vi "Create Init File.vi"(8 "error in (no error)":errorcluster caption="entrée d'erreur (pas d'erreur)", 9 "Nom du fichier ini":string, 10 "Répertoire de l'appli":path, 11 "Container en entrée":refnum<class "Container.lvclass">) -> (0 "error out":errorcluster caption="sortie d'erreur", 2 "Répertoire fichier ini out":path, 3 "Container en sortie":refnum<class "Container.lvclass">)   [LabVIEW 2023, in "Container.lvclass"]
uses:
  Container.lvclass
  Container.lvclass/Container.ctl
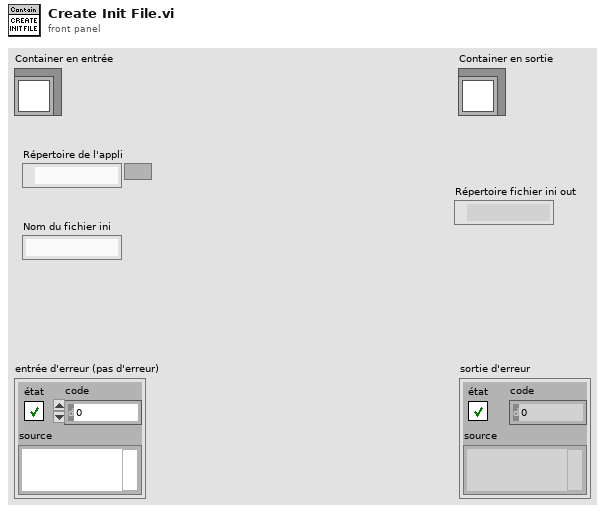
[diagram p1: front panel]
types:
  T1 = enum16{"open", "replace", "create", "open or create", "replace or create", "replace or create with confirmation"}
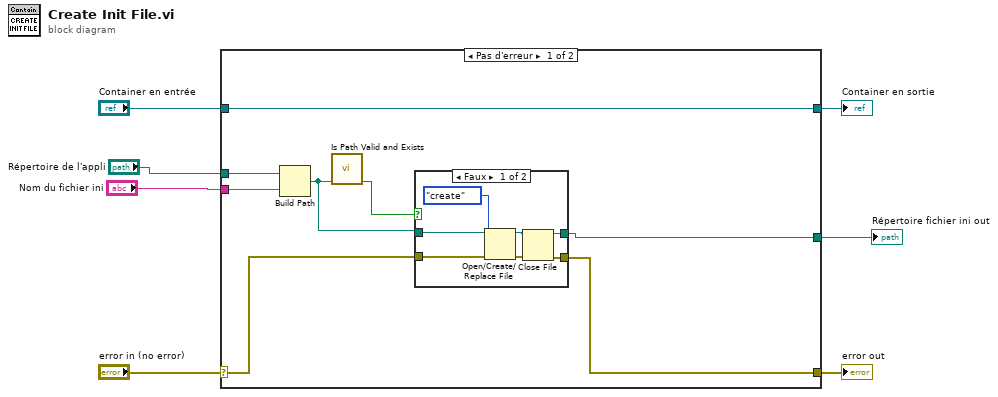
[diagram p0: block diagram]
diagram:
  n1 = case shown="Pas d'erreur" "error in (no error)" {
    selector: "error in (no error)" -> [w10 w26]
    tunnel: [w8 w26] -> w6
    tunnel: [w15 w25] -> w4
    tunnel: "Container en entrée" -> [w15 w25]
    tunnel: "Répertoire de l'appli" -> [w12 _]
    tunnel: "Nom du fichier ini" -> [w11 _]
    tunnel: [w9 _] -> w1
    frame No Error {
      n2 = Build Path(base path=w12, name or relative path=w11) -> (appended path=w13:path)
      n3 = call <userlib>:"Is Path Valid and Exists.vi"("File/Folder Path"=w13) -> ("Valid and Exists?"=w14:bool)  [unwired: 9 in, 1 out]
      n4 = case "Structure Condition" shown="Faux" w14 {
        tunnel: [w20 w24] -> w9
        tunnel: w13 -> [w22 w24]
        tunnel: w10 -> [w18 w23]
        tunnel: [w16 w23] -> w8
        frame False {
          n5 = Open/Create/Replace File(file path (use dialog)=w22, error in=w18, operation (0:open)=T1."create" ("opération (0 : open)")) -> (refnum out=w21:refnum<file>, error out=w17:errorcluster)  [unwired: 3 in, 1 out]
          n6 = Close File(refnum=w21, error in=w17) -> (path=w20:path, error out=w16:errorcluster)
        }
        frame True {
        }
      }
    }
    frame Error {
    }
  }
  "error out" <- w6
  "Container en sortie" <- w4
  "Répertoire fichier ini out" <- w1
